vi "Motion Profile Right Drive Control.vi"(10 "Start Motion Profile?":bool, 11 "Cluster In":T11) -> (3 "Cluster Out":T11)   [LabVIEW 2018]
uses:
  <vilib>/Rock Robotics/WPI/MotorControl/WPI_MotorControlDeviceRef.ctl
  <vilib>/Rock Robotics/WPI/MotorControl/WPI_MotorControlType.ctl
  <vilib>/Rock Robotics/SystemInterfaces/DIO/FPGA_DIOPWMChannel.ctl
  <vilib>/Rock Robotics/WPI/PWM/WPI_PWMDeadband.ctl
  <vilib>/Rock Robotics/SystemInterfaces/DIO/FPGA_DIOChannel.ctl
  <vilib>/Rock Robotics/WPI/Joystick/WPI_JoystickDevRef.ctl
  <vilib>/Rock Robotics/WPI/Joystick/WPI_JoystickDeviceEnum.ctl
  <vilib>/Rock Robotics/WPI/DriverStation/WPI_DriverStationRobotMode2.ctl
  <vilib>/Rock Robotics/WPI/RobotDrive/WPI_RobotDriveDevRef.ctl
  Vision States.ctl
  <vilib>/Rock Robotics/WPI/ThirdParty/Phoenix-LabVIEW/Motor Controller/Controls/CTRE_Phoenix_MotorControl_MotionProfileControlMode.ctl
  Robot Global Data.vi
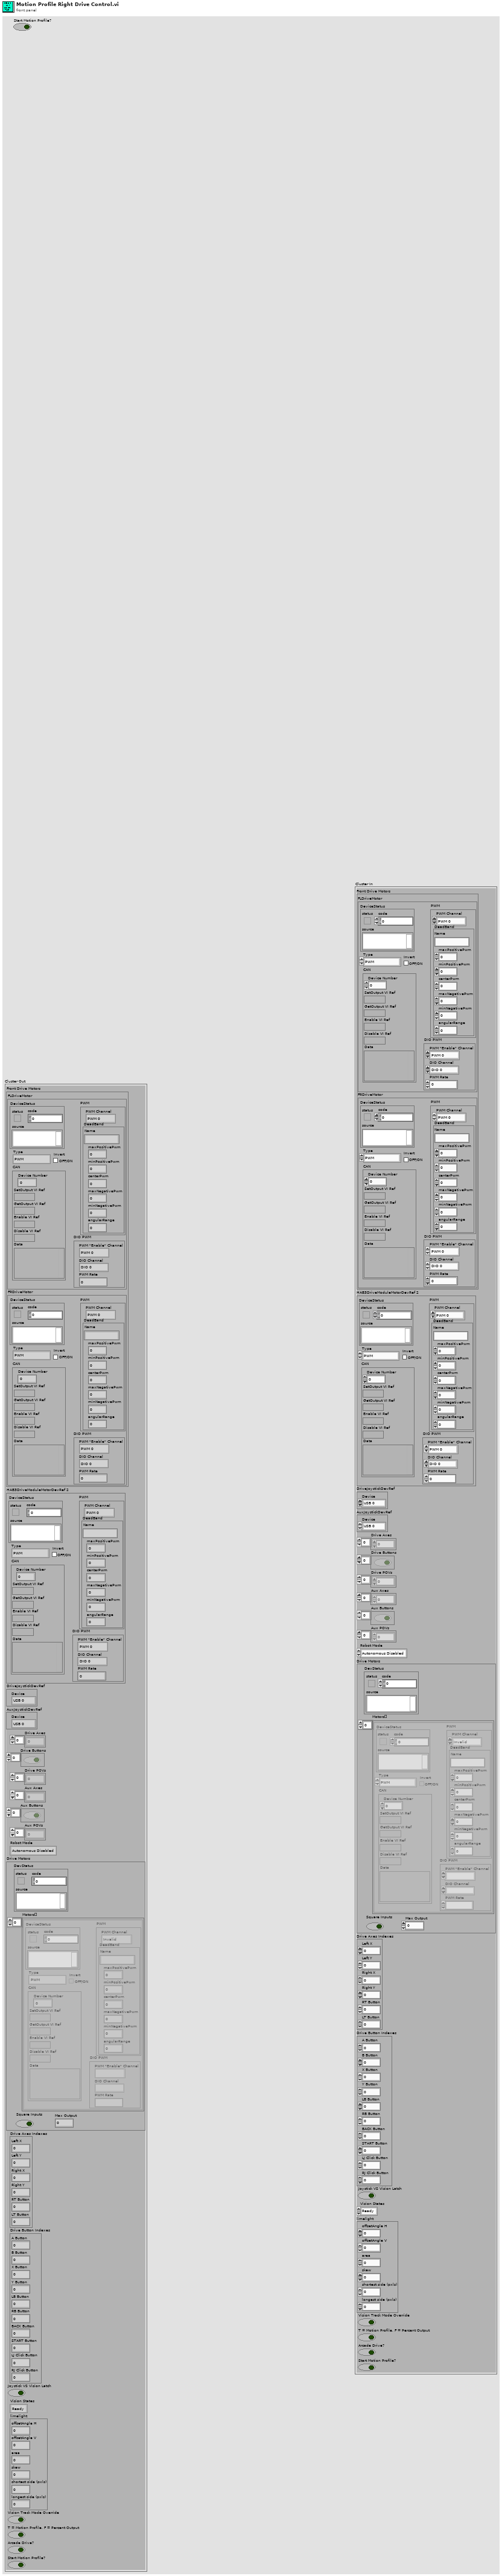
[diagram p1: front panel]
types:
  T1 = typedef "WPI_MotorControlDeviceRef.ctl" = cluster{"DeviceStatus":errorcluster, "Type":T2, "PWM":cluster{"PWM Channel":T3, "DeadBand":T4}, "CAN":cluster{"Device Number":u8, "SetOutput VI Ref":variant, "GetOutput VI Ref":variant, "Enable VI Ref":variant, "Disable VI Ref":variant, "Data":variant}, "Invert":bool, "DIO PWM":cluster{"PWM \"Enable\" Channel":T3, "DIOChannel":T5, "PWM Rate":dbl}}
  T2 = typedef "WPI_MotorControlType.ctl" = enum16{"PWM", "CAN", "DIO PWM"}
  T3 = typedef "FPGA_DIOPWMChannel.ctl" = enum8{"PWM 0", "PWM 1", "PWM 2", "PWM 3", "PWM 4", "PWM 5", "PWM 6", "PWM 7", "PWM 8", "PWM 9", "PWM MXP 0", "PWM MXP 1", "PWM MXP 2", "PWM MXP 3", "PWM MXP 4", "PWM MXP 5", "PWM MXP 6", "PWM MXP 7", "PWM MXP 8", "PWM MXP 9", "Invalid"}
  T4 = typedef "WPI_PWMDeadband.ctl" = cluster{"Name":string, "maxPositivePwm":i32, "minPositivePwm":i32, "centerPwm":i32, "maxNegativePwm":i32, "minNegativePwm":i32, "angularRange":u16}
  T5 = typedef "FPGA_DIOChannel.ctl" = enum8{"DIO 0", "DIO 1", "DIO 2", "DIO 3", "DIO 4", "DIO 5", "DIO 6", "DIO 7", "DIO 8", "DIO 9", "DIO MXP 0", "DIO MXP 1", "DIO MXP 2", "DIO MXP 3", "DIO MXP 4", "DIO MXP 5", "DIO MXP 6", "DIO MXP 7", "DIO MXP 8", "DIO MXP 9", "DIO MXP 10", "DIO MXP 11", "DIO MXP 12", "DIO MXP 13", "DIO MXP 14", "DIO MXP 15", "SPI Port CS1", "SPI Port CS2", "SPI Port CS3", "SPI Port MISO", "SPI Port MOSI", "Invalid"}
  T6 = typedef "WPI_JoystickDevRef.ctl" = cluster{"Device":T7}
  T7 = typedef "WPI_JoystickDeviceEnum.ctl" = enum16{"USB 0", "USB 1", "USB 2", "USB 3", "USB 4", "USB 5"}
  T8 = typedef "WPI_DriverStationRobotMode2.ctl" = enum16{"Autonomous Disabled", "Autonomous Enabled", "Teleop Disabled", "Teleop Enabled", "Disconnected", "Finish", "Test Disabled", "Test Enabled", "Emergency Stopped"}
  T9 = typedef "WPI_RobotDriveDevRef.ctl" = cluster{"DevStatus":errorcluster, "Motors[]":T1[], "Square Inputs":bool, "Max Output":dbl}
  T10 = typedef "Vision States.ctl" = enum16{"Ready", "Forward Until Target at Edge", "Vision Track"}
  T11 = cluster{"Front Drive Motors":cluster{"FLDriveMotor":T1, "FRDriveMotor":T1}, "HAB3DriveModuleMotorDevRef 2":T1, "DriveJoystickDevRef":T6, "AuxJoystickDevRef":T6, "Drive Axes":dbl[], "Drive Buttons":bool[], "Drive POVs":i16[], "Aux Axes":dbl[], "Aux Buttons":bool[], "Aux POVs":i16[], "Robot Mode":T8, "Drive Motors":T9, "Drive Axes Indexes":cluster{"Left X":i32, "Left Y":i32, "Right X":i32, "Right Y":i32, "RT Button":i32, "LT Button":i32}, "Drive Button Indexes":cluster{"A Button":i32, "B Button":i32, "X Button":i32, "Y Button":i32, "LB Button":i32, "RB Button":i32, "BACK Button":i32, "START Button":i32, "LJ Click Button":i32, "RJ Click Button":i32}, "Joystick VS Vision Latch":bool, "Vision States":T10, "limelight":cluster{"offsetAngle H":dbl, "offsetAngle V":dbl, "area":dbl, "skew":dbl, "shortest side (pxls)":dbl, "longest side (pxls)":dbl}, "Vision Track Mode Override":bool, "T = Motion Profile, F = Percent Output":bool, "Arcade Drive?":bool, "Start Motion Profile?":bool}
  T12 = cluster{"Top Buffer Remaining":i32, "Top Buffer Count":i32, "Bottom Buffer Count":i32, "Has Underrun?":bool, "Is Underrun?":bool, "Active Point Valid?":bool, "Is Last?":bool, "Profile Slot Select 0":i32, "Output Enable":i32, "Time Duration (ms)":i32, "Profile Slot Select 1":i32}
  T13 = typedef "CTRE_Phoenix_MotorControl_MotionProfileControlMode.ctl" = u16
  T14 = typedef "CTRE_Phoenix_MotorControl_BufferedTrajectoryPointStream_DeviceRef.ctl" = cluster{"Handle":u64, "Library Path":path}
  T15 = cluster{"Mot Prof Active Velocity":dbl, "Mot Prof Active Position":dbl, "Mot Prof  Is Under Run":bool, "Mot Prof  Has Under Run":bool, "Mot Prof Active Is Last":bool, "Mot Prof Active Is Valid":bool, "Top Mot Prof Count":i32, "Btm Mot Prof Count":i32, "Is Motion Profile Finished?":bool}
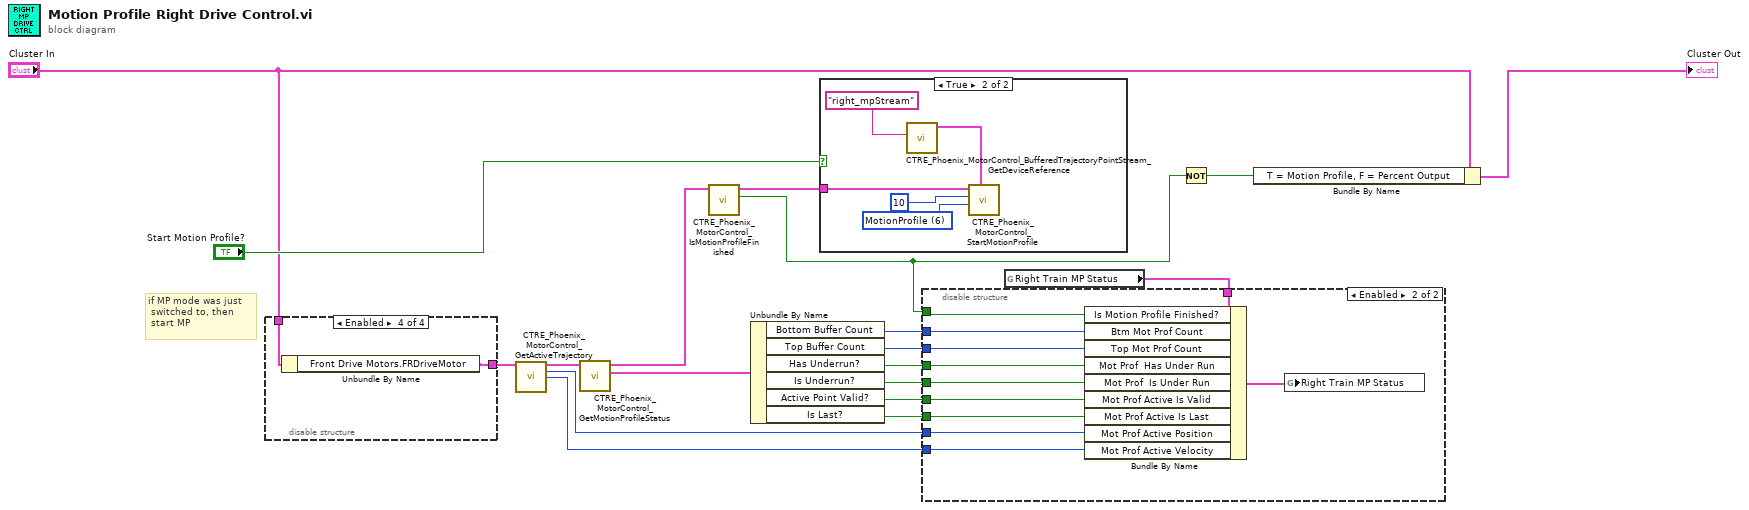
[diagram p0: block diagram]
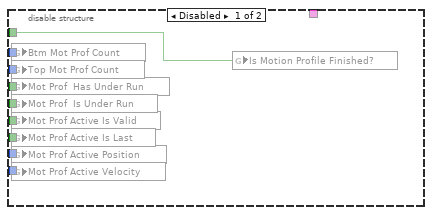
[diagram p2: hidden frame]
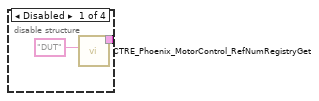
[diagram p3: hidden frame]
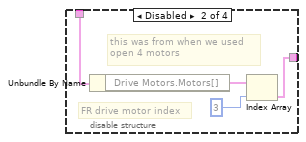
[diagram p4: hidden frame]
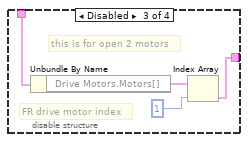
[diagram p5: hidden frame]
diagram:
  # "if MP mode was just\n switched to, then\n start MP"
  n1 = disable-structure shown="Enabled" {
    disable-tunnel: [w21 w24 w27 w30] -> w17
    disable-tunnel: "Cluster In" -> [_ w25 w26 w31]
    frame Disabled {
      n2 = call <vilib>:"CTRE_Phoenix_MotorControl_RefNumRegistryGet.vi"("refnum name"="DUT") -> ("PhoenixMotorControlDevRef"=w21:T1)  [unwired: 9 in, 1 out]
    }
    frame Disabled {
      # "this was from when we used\nopen 4 motors"
      # "FR drive motor index"
      n3 = Unbundle By Name(w25) -> ("Drive Motors.Motors[]"=w23:T1[])
      n4 = Index Array(array=w23, index=3) -> (element=w24:T1)
    }
    frame Disabled {
      # "this is for open 2 motors"
      # "FR drive motor index"
      n5 = Unbundle By Name(w26) -> ("Drive Motors.Motors[]"=w29:T1[])
      n6 = Index Array(array=w29, index=1) -> (element=w27:T1)
    }
    frame Enabled {
      n7 = Unbundle By Name(w31) -> ("Front Drive Motors.FRDriveMotor"=w30:T1)
    }
  }
  n8 = call <vilib>:"CTRE_Phoenix_MotorControl_GetActiveTrajectory.vi"("PhoenixMotorControlDevRef"=w17) -> ("PhoenixMotorControlDevRef"=w15:T1, "Position (Sensor Units)"=w4:i32, "Velocity (Sensor Units per 100 ms)"=w3:i32)  [unwired: 10 in, 2 out]
  n9 = call <vilib>:"CTRE_Phoenix_MotorControl_GetMotionProfileStatus.vi"("PhoenixMotorControlDevRef"=w15) -> ("Motion Profile Status"=w16:T12, "PhoenixMotorControlDevRef"=w14:T1)  [unwired: 8 in, 1 out]
  n10 = call <vilib>:"CTRE_Phoenix_MotorControl_IsMotionProfileFinished.vi"("PhoenixMotorControlDevRef"=w14) -> ("Is Motion Profile Finished?"=w11:bool, "PhoenixMotorControlDevRef"=w13:T1)  [unwired: 8 in, 1 out]
  n11 = Unbundle By Name(w16) -> ("Bottom Buffer Count"=w10:i32, "Top Buffer Count"=w9:i32, "Has Underrun?"=w8:bool, "Is Underrun?"=w7:bool, "Active Point Valid?"=w6:bool, "Is Last?"=w5:bool)
  n12 = case shown="True" "Start Motion Profile?" {
    tunnel: w13 -> [_ w36]
    frame False {
    }
    frame True {
      w35 = T13 6 items=["MotionProfile"=6, "MotionProfileArc"=10] ("Control Mode")
      n13 = call <vilib>:"CTRE_Phoenix_MotorControl_BufferedTrajectoryPointStream_GetDeviceReference.vi"("refnum name"="right_mpStream") -> ("BufferedTrajectoryPointStream_DevRef"=w32:T14)  [unwired: 9 in, 1 out]
      n14 = call <vilib>:"CTRE_Phoenix_MotorControl_StartMotionProfile.vi"("BufferedTrajectoryPointStream_DevRef"=w32, "Control Mode"=w35, "minBufferedPts"=u32 10, "PhoenixMotorControlDevRef"=w36) -> ()  [unwired: 6 in, 2 out]
    }
  }
  n15 = global read "Robot Global Data.vi" "Right Train MP Status"() -> (w12:T15)
  n16 = disable-structure shown="Enabled" {
    disable-tunnel: w3 -> [w45 w53]
    disable-tunnel: w4 -> [w44 w54]
    disable-tunnel: w5 -> [w43 w47]
    disable-tunnel: w6 -> [w42 w48]
    disable-tunnel: w7 -> [w41 w49]
    disable-tunnel: w8 -> [w40 w50]
    disable-tunnel: w9 -> [w39 w55]
    disable-tunnel: w10 -> [w38 w56]
    disable-tunnel: w11 -> [w37 w52]
    disable-tunnel: w12 -> [_ w51]
    frame Disabled {
      n17 = global write "Robot Global Data.vi" "Btm Mot Prof Count"(w38) -> ()
      n18 = global write "Robot Global Data.vi" "Top Mot Prof Count"(w39) -> ()
      n19 = global write "Robot Global Data.vi" "Mot Prof  Has Under Run"(w40) -> ()
      n20 = global write "Robot Global Data.vi" "Mot Prof  Is Under Run"(w41) -> ()
      n21 = global write "Robot Global Data.vi" "Mot Prof Active Is Valid"(w42) -> ()
      n22 = global write "Robot Global Data.vi" "Mot Prof Active Is Last"(w43) -> ()
      n23 = global write "Robot Global Data.vi" "Mot Prof Active Position"(w44) -> ()
      n24 = global write "Robot Global Data.vi" "Mot Prof Active Velocity"(w45) -> ()
      n25 = global write "Robot Global Data.vi" "Is Motion Profile Finished?"(w37) -> ()
    }
    frame Enabled {
      n26 = Bundle By Name(cluster=w51, "Is Motion Profile Finished?"=w52, "Btm Mot Prof Count"=w56, "Top Mot Prof Count"=w55, "Mot Prof  Has Under Run"=w50, "Mot Prof  Is Under Run"=w49, "Mot Prof Active Is Valid"=w48, "Mot Prof Active Is Last"=w47, "Mot Prof Active Position"=w54, "Mot Prof Active Velocity"=w53) -> (w46:T15)
      n27 = global write "Robot Global Data.vi" "Right Train MP Status"(w46) -> ()
    }
  }
  n28 = Not(x=w11) -> (.not. x?=w19:bool)
  n29 = Bundle By Name(cluster="Cluster In", "T = Motion Profile, F = Percent Output"=w19) -> (→"Cluster Out":T11)
